vi "Write Data to TDMS File.vi"(7 "TDMS File Path":path, 8 "error in (no error)":errorcluster, 10 "Attributes":T1, 11 "Waveforms":waveform(sgl)[](array[waveform])) -> (0 "error out":errorcluster)   [LabVIEW 2013]
doc: "Statnett PMU Reference Library\nWrites Data To TDMS File"
panel:
  # "INPUT"
  # "INTERMEDIATE"
  # "OUTPUT"
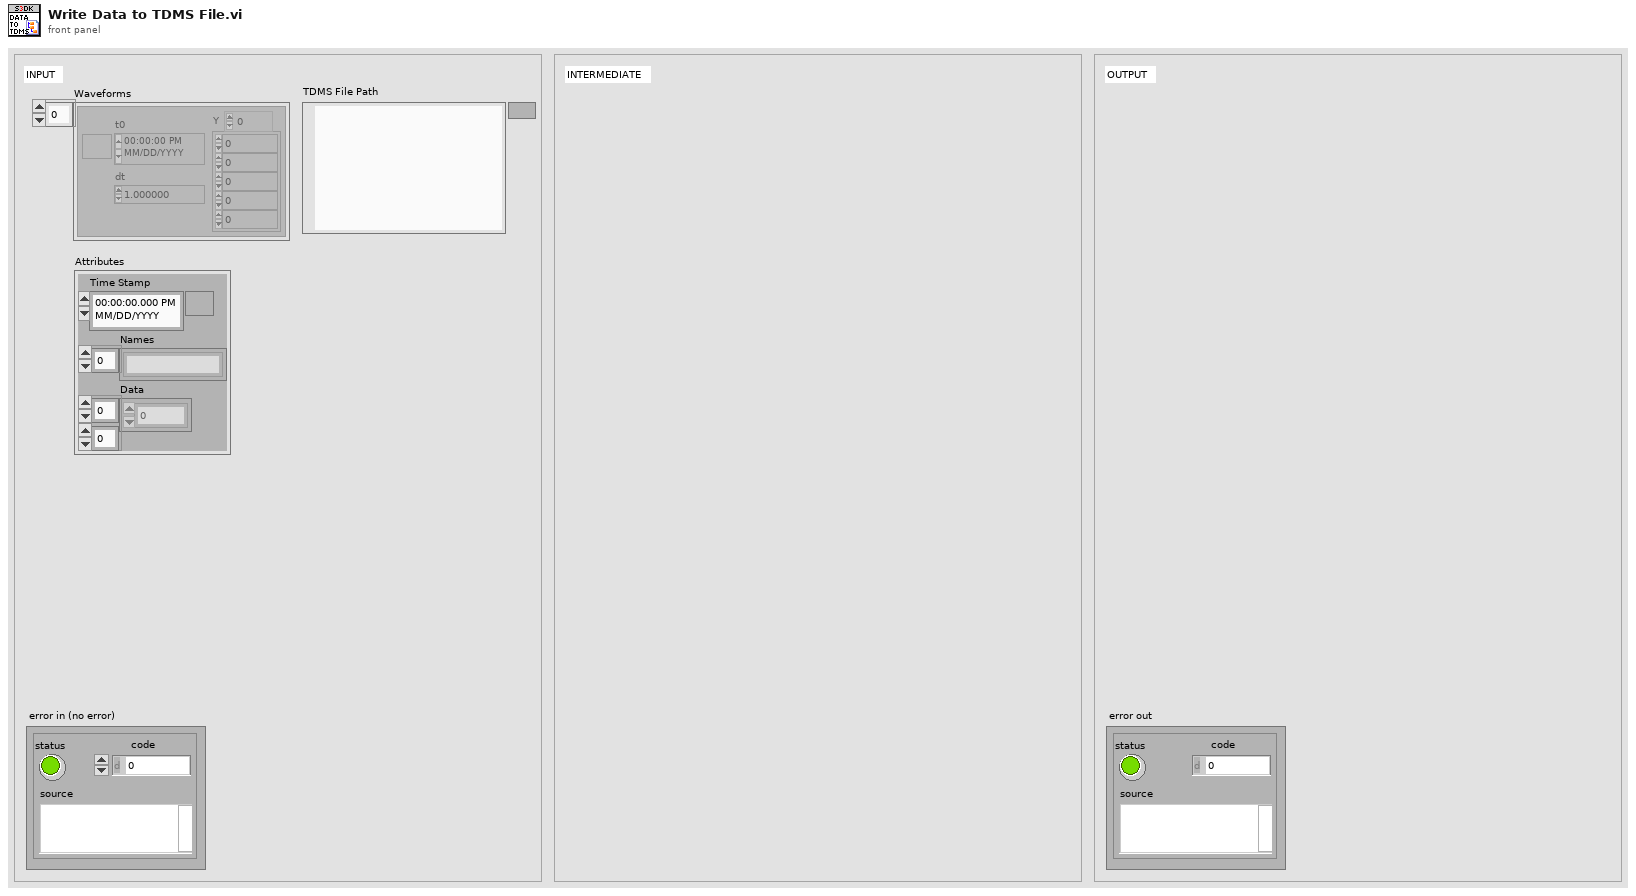
[diagram p1: front panel]
types:
  T1 = cluster{"Time Stamp":timestamp, "Names":string[], "Data":dbl[][]}
  T2 = enum16{"open", "open or create", "create or replace", "create", "open (read-only)"}
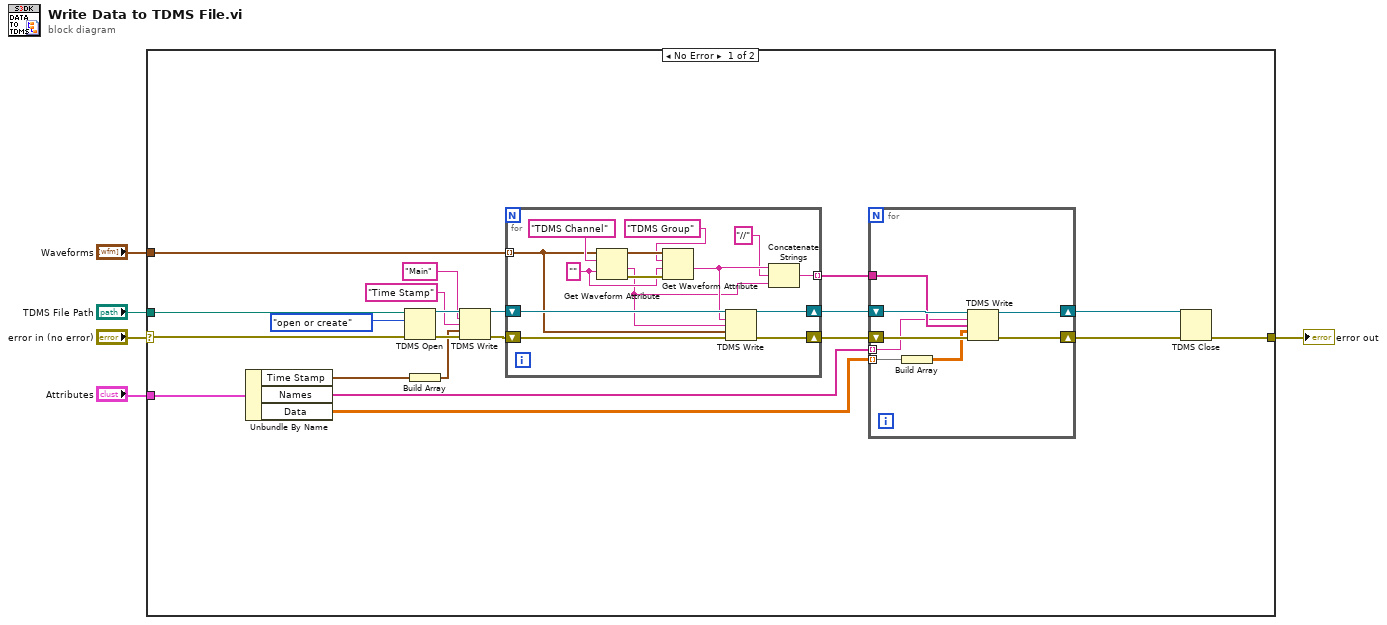
[diagram p0: block diagram]
diagram:
  n1 = case shown="No Error" "error in (no error)" {
    selector: "error in (no error)" -> [w7 w49]
    tunnel: [w6 w49] -> w4
    tunnel: "TDMS File Path" -> [w10 _]
    tunnel: "Attributes" -> [w9 _]
    tunnel: "Waveforms" -> [w8 _]
    frame No Error {
      n2 = Unbundle By Name(w9) -> ("Time Stamp"=w20:timestamp, "Names"=w14:string[], "Data"=w13:dbl[][])
      n3 = TDMS Open(8:w7, 10:T2."open or create" ("operation (0:open)"), 11:w10) -> (0:w24:errorcluster, 3:w25:refnum<k34>)  [unwired: 4 in]
      n4 = Build Array(w20) -> (w21:timestamp[])
      n5 = TDMS Write(0:w25, 5:"Main" ("group name in (Untitled)"), 7:"Time Stamp" ("group name in (Untitled)"), 9:w21, 11:w24) -> (4:w19:refnum<k34>, 15:w18:errorcluster)  [unwired: 1 in, 2 out]
      n6 = for {
        tunnel: w8 -> [w34] mode=indexing
        shift-right: [w31] -> w16
        shift-left: w19 -> [w35]
        shift-right: [w32] -> w15
        shift-left: w18 -> [w33]
        tunnel: [w27] -> w17 mode=indexing
        w36 = "" ("name")
        n7 = Get Waveform Attribute(5:w36, 6:"TDMS Channel" ("name"), 7:w34) -> (0:w38:errorcluster, 1:w29:string, 3:w39:waveform(sgl))  [unwired: 1 in, 1 out]
        n8 = Get Waveform Attribute(4:w38, 5:w36, 6:"TDMS Group" ("name"), 7:w39) -> (1:w30:string)  [unwired: 3 out]
        n9 = TDMS Write(0:w35, 5:w30, 7:w29, 9:w34, 11:w33) -> (4:w31:refnum<k34>, 15:w32:errorcluster)  [unwired: 1 in, 2 out]
        n10 = Concatenate Strings(w30, "//" ("string"), w29) -> (w27:string)
      }
      n11 = for {
        shift-right: [w48] -> w12
        shift-left: w16 -> [w46]
        shift-right: [w47] -> w11
        shift-left: w15 -> [w45]
        tunnel: w17 -> [w42]
        tunnel: w14 -> [w41] mode=indexing
        tunnel: w13 -> [w44] mode=indexing
        n12 = Build Array(w44) -> (w43:dbl[][])
        n13 = TDMS Write(0:w46, 5:w41, 7:w42, 9:w43, 11:w45) -> (4:w48:refnum<k34>, 15:w47:errorcluster)  [unwired: 1 in, 2 out]
      }
      n14 = TDMS Close(8:w11, 11:w12) -> (0:w6:errorcluster)  [unwired: 1 out]
    }
    frame Error {
    }
  }
  "error out" <- w4
